vi "ATS_ID.vi"() -> (1 "Found":bool, 2 "ATS_System":cluster{"System":u32, "Devices":T1[]}[](array[cluster]), 3 "#System":i32)   [LabVIEW 2015]
doc: "_____AlazarTech, Scope_____\n\nIdentify ALL System and there boards.\n\nOutput:\n\"ATS_System\" = systems identified\n : System = System ID\n : Handle = communication refnum\n : Board = identification\n : CPLD = version of the device software.\n : MemorySize = size of the memory on the board in bytes.\n : SampleSize = number of bit of the digitizer."
uses:
  ATS_ctl/Device_Info.ctl
  ATS_ctl/ATS_Cards_GBL.vi
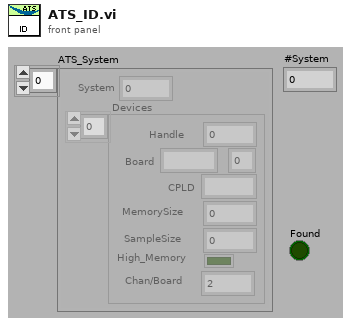
[diagram p1: front panel]
types:
  T1 = typedef "Device_Info.ctl" = cluster{"Handle":u32, "Board":string, "CPLD":string, "MemorySize":u32, "SampleSize":u8, "ID":i32, "High_Memory":bool, "Chan/Board":u8}
  T2 = typedef "ATS_Global_Specs_Ctrl.ctl" = cluster{"ClckSource":cluster{"Internal":bool, "External":bool, "Medium Ext.":bool, "Slow Ext.":bool, "Ext. AC":bool, "Ext. DC":bool, "Ext. (PLL)":bool}, "ClckRate":cluster{"1 kS/s":bool, "2 kS/s":bool, "5 kS/s":bool, "10 kS/s":bool, "20 kS/s":bool, "50 kS/s":bool, "100 kS/s":bool, "200 kS/s":bool, "500 kS/s":bool, "1 MS/s":bool, "2 MS/s":bool, "5 MS/s":bool, "10 MS/s":bool, "20 MS/s":bool, "25 MS/s":bool, "50 MS/s":bool, "100 MS/s":bool, "125 MS/s":bool, "160 MS/s":bool, "180 MS/s":bool, "200 MS/s":bool, "250 MS/s":bool, "500 MS/s":bool, "1 GS/s":bool}, "ClckEdge":cluster{"Rising":bool, "Falling":bool}, "InputCoupling":cluster{"AC":bool, "DC":bool}, "InputRange":cluster{"20mV":bool, "40mV":bool, "50mV":bool, "80mV":bool, "100mV":bool, "200mV":bool, "400mV":bool, "500mV":bool, "800mV":bool, "1 V":bool, "2 V":bool, "4 V":bool, "5 V":bool, "8 V":bool, "10 V":bool, "16 V":bool, "20 V":bool, "40 V":bool, "HiFi":bool, "1.25 V":bool}, "Impedance":cluster{"1M ohms":bool, "50 ohms":bool, "300 ohms":bool}, "Bandwidth":cluster{"Full":bool, "Reduce":bool}, "RangeLim(50)":string, "AsyncDMA":cluster{"OnBoard":bool, "FPGA":bool}, "Memory":cluster{"VerifMem":bool, "HighMem":bool, "Combine":bool, "HighRecord":bool}, "ExtTrigCoupling":cluster{"AC":bool, "DC":bool}, "ExtTrigRange":cluster{"1 V":bool, "5 V":bool, "\nTTL":bool}, "AUX_IO_Trig":cluster{"Trig_Out":bool, "Trig_In":bool}, "AUX_IO_Slope":cluster{"Rising":bool, "Falling":bool}, "MaxPretrig":cluster{"MEM":u32, "FIFO":u32}, "AUX_I/O_Trig":cluster{"OUT_Trigger":bool, "OUT_PACER":bool, "OUT_BUSY":bool, "OUT_CLOCK":bool, "OUT_RESERVED":bool, "OUT_CAPTURE_ALMOST_DONE":bool, "OUT_AUXILIARY":bool, "OUT_SERIAL_DATA":bool, "IN_TRIGGER_ENABLE":bool, "IN_DIGITAL_TRIGGER":bool, "IN_GATE":bool, "IN_CAPTURE_ON_DEMAND":bool, "IN_RESET_TIMESTAMP":bool, "IN_SLOW_EXTERNAL_CLOCK":bool, "INPUT_AUXILIARY":bool, "INPUT_SERIAL_DATA":bool}, "ChannelsPerBoard":u8}
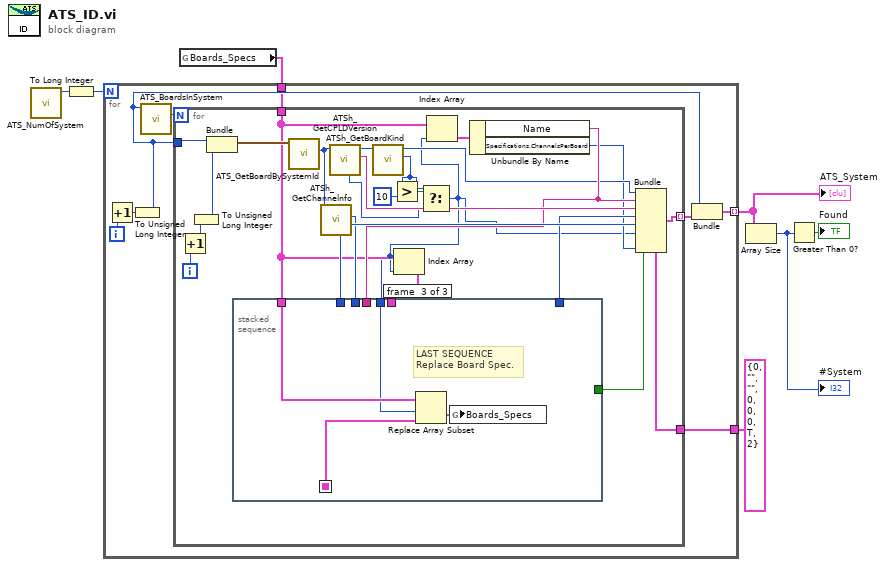
[diagram p0: block diagram]
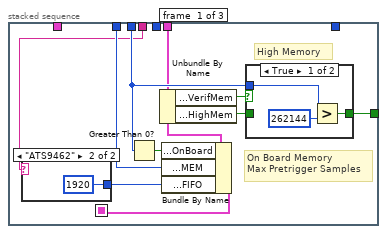
[diagram p2: hidden frame]
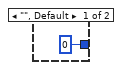
[diagram p3: hidden frame]
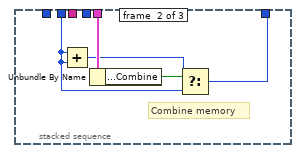
[diagram p5: hidden frame]
diagram:
  n1 = call "ATS_NumOfSystem.vi"() -> ("Num_Of_System"=w7:u32)  [unwired: 7 in]
  n2 = To Long Integer(number=w7) -> (32bit integer=w2:i32)
  n3 = global read "ATS_Cards_GBL.vi" "Boards_Specs"() -> (w1:cluster{"Name":string, "Specifications":T2}[])
  n4 = for {
    N: w2 -> [_]
    tunnel: [w10] -> w5 mode=indexing
    tunnel: T1 {"Handle"=0, "Board"="", "CPLD"="", "MemorySize"=0, "SampleSize"=0, "ID"=0, "High_Memory"=TRUE, "Chan/Board"=2} ("DevInfo_In") -> [w12]
    tunnel: w1 -> [w8]
    i -> [w14]
    n5 = Increment(x=w14) -> (x+1=w13:i32)
    n6 = To Unsigned Long Integer(number=w13) -> (unsigned 32bit integer=w9:u32)
    n7 = call "ATS_BoardsInSystem.vi"("sid_In"=w9) -> ("Num_Of_Boards"=w15:u32)  [unwired: 5 in, 1 out]
    n8 = for {
      N: w15 -> [_]
      tunnel: w9 -> [w35]
      tunnel: [w36] -> w11 mode=indexing
      tunnel: w12 -> [w39]
      tunnel: w8 -> [w22]
      i -> [w41]
      n9 = Increment(x=w41) -> (x+1=w40:i32)
      n10 = To Unsigned Long Integer(number=w40) -> (unsigned 32bit integer=w34:u32)
      n11 = Bundle(w35, w34) -> (w33:cluster{u32, u32})  [unwired: 1 in]
      n12 = call "ATS_GetBoardBySystemId.vi"("Sys/Board_In"=w33) -> ("Handle"=w24:u32)  [unwired: 5 in, 1 out]
      n13 = call "ATSh_GetChannelnfo.vi"("HandleIn"=w24) -> ("SampleSize"=w37:u8, "MemSize/Channel(Sample)"=w32:u32, "MaxPretriggerSamples"=w28:u32)  [unwired: 6 in, 2 out]
      n14 = call "ATSh_GetCPLDVersion.vi"("HandleIn"=w24) -> ("Version"=w38:string, "HandleOut"=w27:u32, "ID"=w17:i32)  [unwired: 6 in, 2 out]
      n15 = call "ATSh_GetBoardKind.vi"("HandleIn"=w27) -> ("ID"=w16:i32, "HandleOut"=w23:u32)  [unwired: 9 in]
      n16 = Greater?(x=w16, y=10) -> (0:w19:bool)
      n17 = Select(t=w16, s=w19, f=w17) -> (s? t:f=w18:i32)
      n18 = Index Array(array=w22, index=w18) -> (element=w30:cluster{"Name":string, "Specifications":T2})
      n19 = Index Array(array=w22, index=w18) -> (element=w26:cluster{"Name":string, "Specifications":T2})
      n20 = Unbundle By Name(w26) -> ("Name"=w25:string, "Specifications.ChannelsPerBoard"=w21:u8)
      n21 = stacked-sequence {
        seq-local: [w45 _ _] -> [_ _ w65]
        tunnel: w32 -> [w47 w60 _]
        tunnel: [w51 _ _] -> w31
        tunnel: w25 -> [w42 _ _]
        tunnel: w30 -> [w46 w62 _]
        tunnel: w22 -> [_ _ w64]
        tunnel: w18 -> [_ _ w63]
        tunnel: [_ w58 _] -> w29
        tunnel: w28 -> [w44 _ _]
        frame #0 {
          # "On Board Memory\nMax Pretrigger Samples"
          # "High Memory"
          n22 = case shown="\"ATS9462\"" w42 {
            tunnel: [u32 0 ("Specifications.MaxPretrig.FIFO") u32 1920 ("Specifications.MaxPretrig.FIFO")] -> w43
            frame "", Default {
            }
            frame "ATS9462" {
            }
          }
          n23 = Greater Than 0?(x=w47) -> (x > 0?=w48:bool)
          n24 = Unbundle By Name(w46) -> ("Specifications.Memory.VerifMem"=w50:bool, "Specifications.Memory.HighMem"=w49:bool)
          n25 = Bundle By Name(cluster=w46, "Specifications.AsyncDMA.OnBoard"=w48, "Specifications.MaxPretrig.MEM"=w44, "Specifications.MaxPretrig.FIFO"=w43) -> (w45:cluster{"Name":string, "Specifications":T2})
          n26 = case shown="True" w50 {
            tunnel: w47 -> [w56 _]
            tunnel: [w54 w57] -> w51
            tunnel: w49 -> [_ w57]
            frame True {
              n27 = Greater?(x=w56, y=u32 262144) -> (0:w54:bool)
            }
            frame False {
            }
          }
        }
        frame #1 {
          # "Combine memory"
          n28 = Add(x=w60, y=w60) -> (x+y=w59:u32)
          n29 = Unbundle By Name(w62) -> ("Specifications.Memory.Combine"=w61:bool)
          n30 = Select(t=w59, s=w61, f=w60) -> (s? t:f=w58:u32)
        }
        frame #2 {
          # "LAST SEQUENCE\nReplace Board Spec."
          n31 = Replace Array Subset(array=w64, new element=w65, index=w63) -> (w66:cluster{"Name":string, "Specifications":T2}[])
          n32 = global write "ATS_Cards_GBL.vi" "Boards_Specs"(w66) -> ()
        }
      }
      n33 = Bundle(cluster=w39, "Handle"=w23, "Board"=w25, "CPLD"=w38, "MemorySize"=w29, "SampleSize"=w37, "ID"=w18, "High_Memory"=w31, "Chan/Board"=w21) -> (w36:T1)
    }
    n34 = Bundle(w9, w11) -> (w10:cluster{u32, T1[]})  [unwired: 1 in]
  }
  "ATS_System" <- w5
  n35 = Array Size(array=w5) -> (size(s)=w4:i32)
  "#System" <- w4
  n36 = Greater Than 0?(x=w4) -> (x > 0?=→"Found":bool)
